vi "Data_Ctrl.vi"() -> ()   [LabVIEW 2019]
uses:
  REV2_Config_Addr.ctl
  <vilib>/event_ctls.llb/eventvkey.ctl
  <vilib>/Instr/_visa.llb/VISA Set IO Buffer Mask.ctl
  <vilib>/Instr/_visa.llb/VISA Flush IO Buffer Mask.ctl
  REV2_Stat_Addr.ctl
  <vilib>/Analysis/1siggen.llb/Ramp Pattern by Samples.vi
  <vilib>/Instr/_visa.llb/VISA Configure Serial Port (Instr).vi
  <vilib>/Analysis/1siggen.llb/Ramp Pattern by Delta.vi
  <vilib>/Analysis/NI_AALBase.lvlib
  <vilib>/ptbypt/NI_PtbyPt.lvlib
panel:
  in  "SAVE":bool
  in  "P0.0002D0.2":bool
  in  "P0.03":bool
  out "VKey":T1
  out "Vbus":dbl(graph)=12.629144668579102
  out "Error count":u64
  out "Array":cluster{"Config Address":T2, dbl}[](array[cluster])=[{"Config Address"=enum."ID", 1.0}, {"Config Address"=enum."Mode", 3.0}, {"Config Address"=enum."Baudrate", 8000000.0}, {"Config Address"=enum."Homing Offset", 0.0}, {"Config Address"=enum."Id P gain", 0.004999999888241291}, {"Config Address"=enum."Id I gain", 0.0010000000474974513}, {"Config Address"=enum."Id D gain", 0.0}, {"Config Address"=enum."Iq P gain", 0.004999999888241291}, {"Config Address"=enum."Iq I gain", 0.0010000000474974513}, {"Config Address"=enum."Iq D gain", 0.0}, {"Config Address"=enum."Velo P gain", 0.4000000059604645}, {"Config Address"=enum."Velo I gain", 0.0010000000474974513}, {"Config Address"=enum."Velo D gain", 0.0}, {"Config Address"=enum."Posi P gain", 0.02500000037252903}, {"Config Address"=enum."Posi I gain", 0.0}, {"Config Address"=enum."Posi D gain", 0.0010000000474974513}, {"Config Address"=enum."DirectForce P", 0.0}, {"Config Address"=enum."DirectForce I", 0.0}, {"Config Address"=enum."DirectForce D", 0.0}, {"Config Address"=enum."Limit Id Max", 50.0}, {"Config Address"=enum."Limit Iq Max", 10.0}, {"Config Address"=enum."Limit Velo Max", 80.0}, {"Config Address"=enum."Limit Posi Min", -131000.0}, {"Config Address"=enum."Limit Posi Max", 131000.0}, {"Config Address"=enum."Voltage Min", 6.0}, {"Config Address"=enum."Voltage Max", 40.0}, {"Config Address"=enum."Low Voltage", 10.0}, {"Config Address"=enum."Temperature Low", 80.0}, {"Config Address"=enum."Temperature High", 100.0}] {"?" format="%#_6f"}
  in  "Read Config":bool
  out "Temperature":cluster{dbl, dbl, dbl}(graph)={25.75, 0.0, 0.0}
  out "ERROR":u8
  out "Iq":cluster{dbl, dbl}(graph)={0.11970416456460953, 0.0}
  out "Id":cluster{dbl, dbl}(graph)={-0.016149107366800308, 0.0}
  out "Theta":cluster{dbl, dbl}(graph)={-51551.1953125, 0.0}
  out "Theta_dot":cluster{dbl, dbl}(graph)={0.09893438220024109, 0.0}
  in  "ID":u8=1
  in  "Read":bool=TRUE
  in  "PID0":bool
  in  "P0.001":bool
  in  "D0.5":bool
  in  "P0.0002":bool
  in  "send sine":bool
  in  "2state":bool
  in  "Chirp":i32(listbox)=2
  out "Waveform Graph":cluster{dbl, dbl, dbl[]}(graph)={0.0, 0.002, array[5500 elements]}
  in  "Sample_rate":dbl=100.0 format="%#_13g"
  out "Theta_LP":sgl=-51551.195
  in  "send chirp":bool
  in  "Enable":bool
  in  "DISABLE":bool
  in  "Write_Mode":bool
  in  "Listbox":i32(listbox)=3
  in  "Write_Limits":bool
  in  "Limits":cluster{"Iq":sgl, "Vel":sgl}={"Iq"=60.0, "Vel"=80.0}
  in  "Goal":T3={"Id"=0.0, "Iq"=0.0, "Posi"=0.0, "Vel"=10.0}
  in  "PID_F":cluster{"P":sgl, "I":sgl, "D":sgl}
  in  "PID_P":cluster{"P":sgl, "I":sgl, "D":sgl}={"P"=0.025, "I"=0.0, "D"=0.001}
  out "Iq":cluster{"Mean":dbl, "Std":dbl}={"Mean"=0.05623460856704041, "Std"=0.04704007521425213} {"Std" format="%.4f"; "Mean" format="%.4f"}
  out "Theta_LP":cluster{"Mean":dbl, "Std":dbl}={"Mean"=-51551.37356875, "Std"=0.30848497864286445}
  out "Id":cluster{"Mean":dbl, "Std":dbl}={"Mean"=0.0007310798299324233, "Std"=0.028296682304707433} {"Std" format="%.4f"; "Mean" format="%.4f"}
  in  "amplitude":dbl=10000.0 format="%#_13g"
  in  "Time":dbl=10.0 format="%#_13g"
  in  "frq_2":dbl=1.0 format="%#_13g"
  in  "frq_1":dbl=1.0 format="%#_13g"
  in  "stop":bool
  in  "Write_Dst":bool
  in  "PID_IqId":cluster{"P":sgl, "I":sgl, "D":sgl}={"P"=0.005, "I"=0.001, "D"=0.0}
  in  "PID_V":cluster{"P":sgl, "I":sgl, "D":sgl}={"P"=0.4, "I"=0.001, "D"=0.0}
  in  "Write_PID":bool
  in  "baud rate":u32=8000000
  in  "Buffer_Size":u32=150000
  in  "VISA resource name":refnum<visa-resource-name>="COM15"
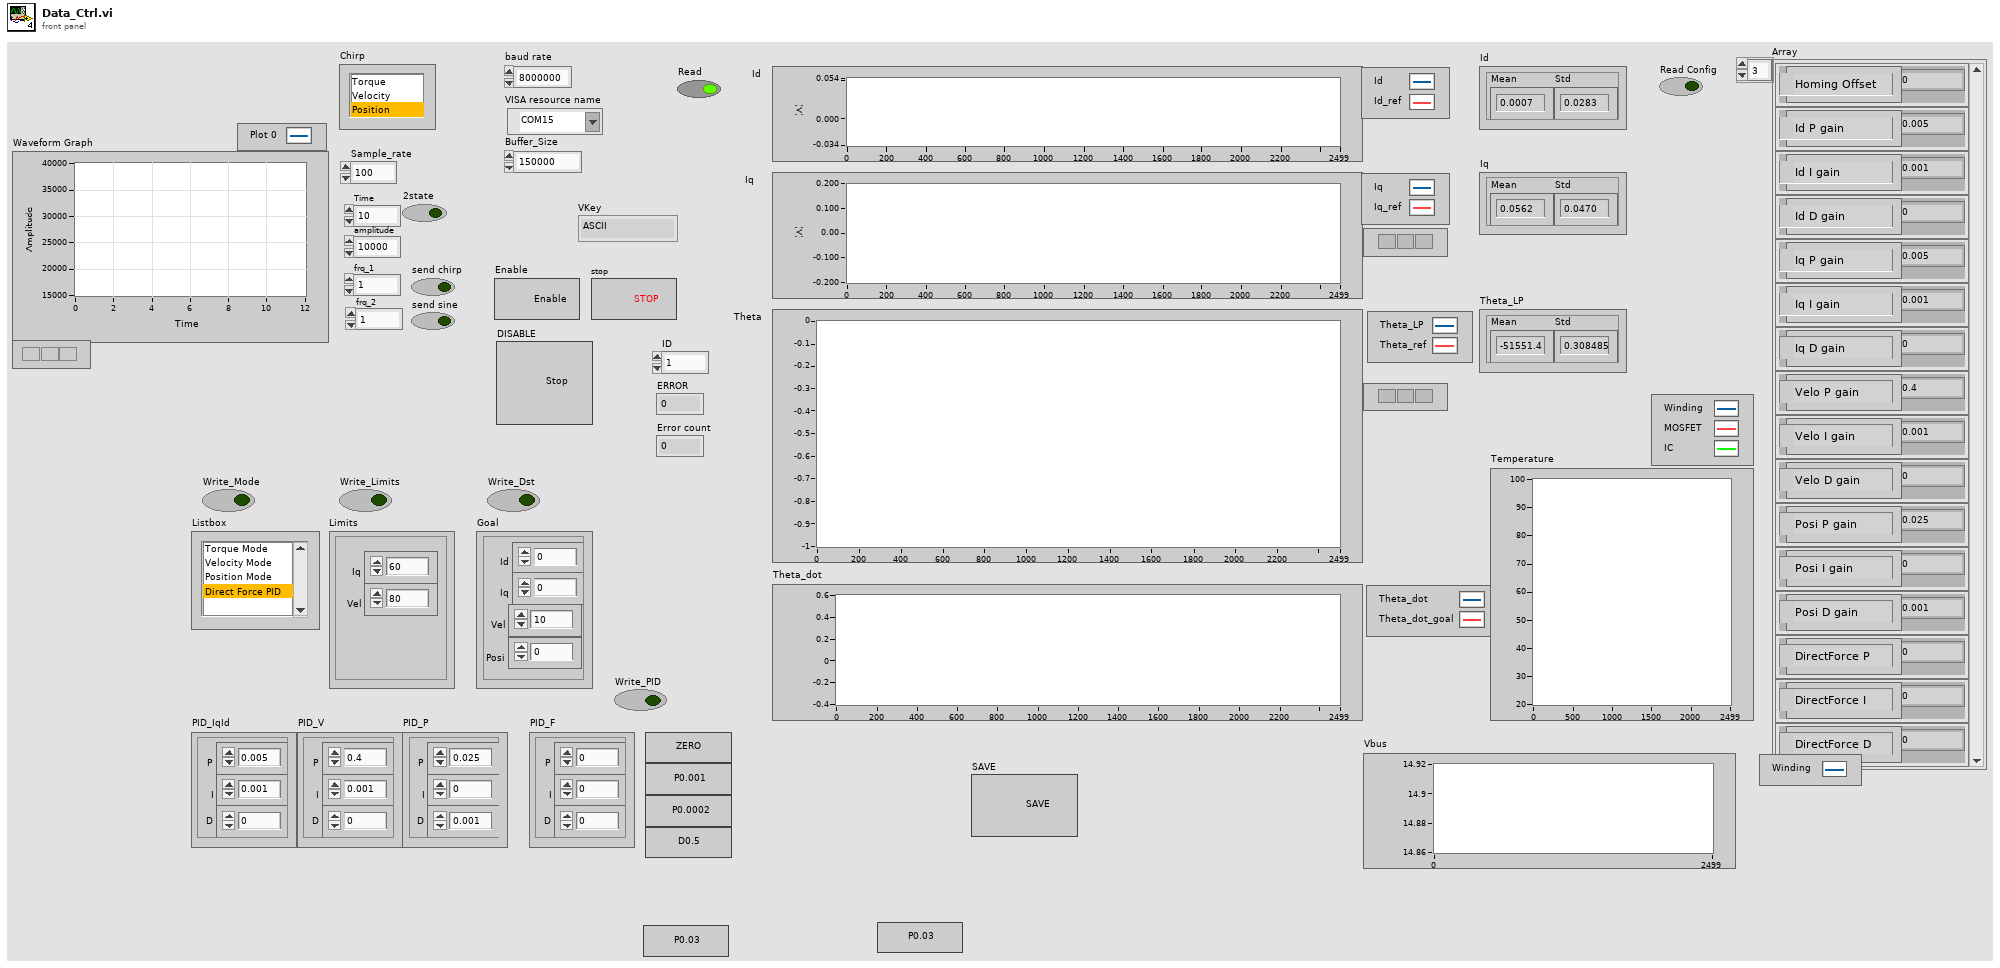
[diagram p1: front panel]
types:
  T1 = typedef "eventvkey.ctl" = enum16{"ASCII", "Enter", "Return", "Shift", "Ctrl", "Alt", "Cmd", "Opt", "Caps", "NumLock", "Clear", "Break", "Up", "Down", "Left", "Right", "Insert", "Delete", "Home", "End", "PageUp", "PageDown", "Escape", "Help", "Pause", "ScrollLock", "F1", "F2", "F3", "F4", "F5", "F6", "F7", "F8", "F9", "F10", "F11", "F12", "F13", "F14", "F15", "F16", "F17", "F18", "F19", "F20", "F21", "F22", "F23", "F24", "Play", "VolumeUp", "VolumeDown", "Mute", "Two Byte Char"}
  T2 = typedef "REV2_Config_Addr.ctl" = enum8{"ID", "Mode", "Baudrate", "Homing Offset", "Id P gain", "Id I gain", "Id D gain", "Iq P gain", "Iq I gain", "Iq D gain", "Velo P gain", "Velo I gain", "Velo D gain", "Posi P gain", "Posi I gain", "Posi D gain", "DirectForce P", "DirectForce I", "DirectForce D", "Limit Id Max", "Limit Iq Max", "Limit Velo Max", "Limit Posi Min", "Limit Posi Max", "Voltage Min", "Voltage Max", "Low Voltage", "Temperature Low", "Temperature High"}
  T3 = cluster{"Id":sgl, "Iq":sgl, "Posi":sgl, "Vel":sgl}
  T4 = typedef "VISA Flush IO Buffer Mask.ctl" = u16
  T5 = typedef "VISA Set IO Buffer Mask.ctl" = u16
  T6 = typedef "REV2_Stat_Addr.ctl" = enum8{"Torque Enable", "Homing Complete", "Goal Id", "Goal Iq", "Goal Velo", "Goal Posi", "Present Id", "Present Iq", "Present Velo", "Present Posi", "Bus Voltage", "Temperature Winding", "Temperature MOSFET", "Temperature IC", "Error Status"}
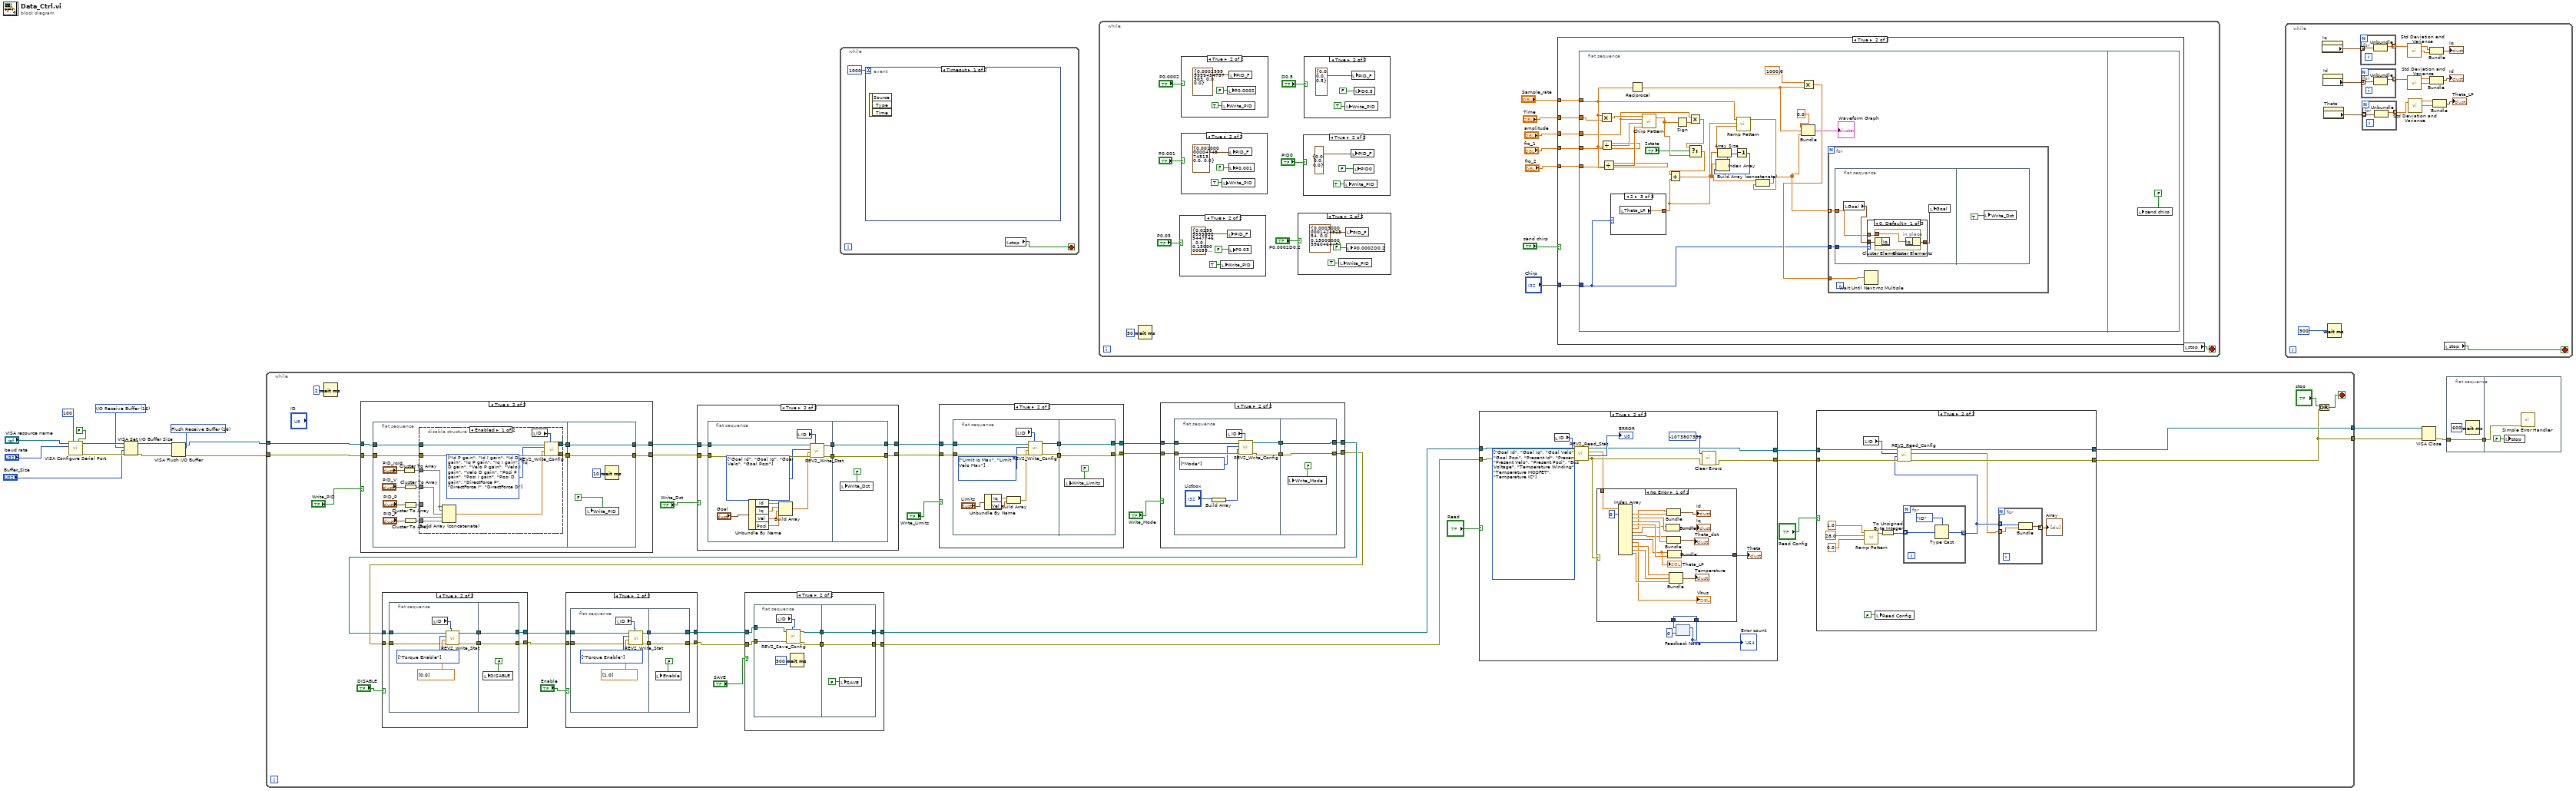
[diagram p0: block diagram]
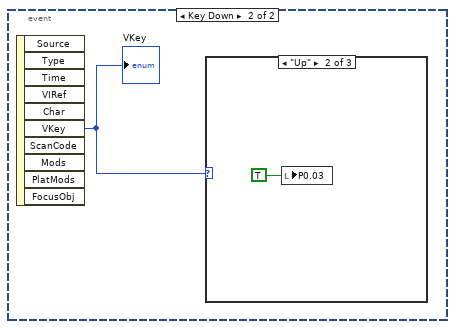
[diagram p2: hidden frame]
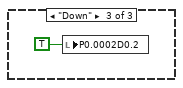
[diagram p4: hidden frame]
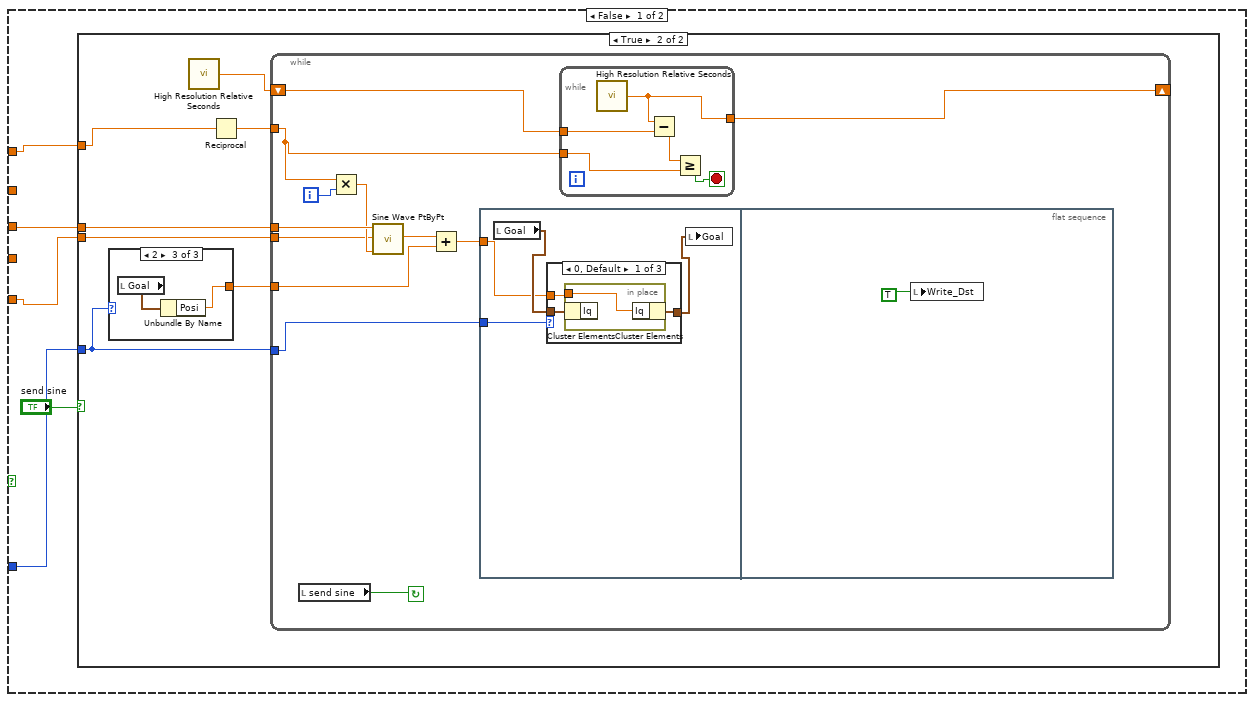
[diagram p11: hidden frame]
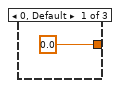
[diagram p13: hidden frame]
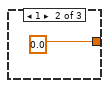
[diagram p14: hidden frame]
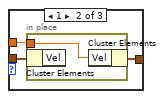
[diagram p15: hidden frame]
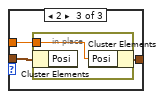
[diagram p16: hidden frame]
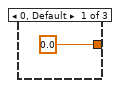
[diagram p17: hidden frame]
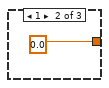
[diagram p18: hidden frame]
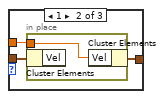
[diagram p19: hidden frame]
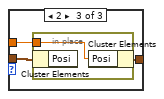
[diagram p20: hidden frame]
diagram:
  w6 = T4 16 items=["Flush Receive Buffer"=16, "Write Transmit Buffer to Device"=32, "Flush Receive Buffer (No I/O)"=64, "Flush Transmit Buffer"=128] ("Mask")
  w10 = T5 16 items=["I/O Receive Buffer"=16, "I/O Transmit Buffer"=32, "I/O Receive and Transmit Buffer"=48] ("Mask")
  n1 = call-poly "VISA Configure Serial Port"("VISA resource name"="VISA resource name", "timeout (10sec)"=u32 100, "Enable Termination\nChar (T)"=FALSE ("Enable Termination\nChar (T)"), "baud rate (9600)"="baud rate") -> ("VISA resource name out"=w12:refnum<visa-resource-name>, "error out"=w11:errorcluster)  [unwired: 10 in]
  n2 = VISA Set I/O Buffer Size(VISA resource name=w12, mask (16)=w10, size (4096)="Buffer_Size", error in (no error)=w11) -> (VISA resource name out=w4:refnum<visa-resource-name>, error out=w5:errorcluster)
  n3 = VISA Flush I/O Buffer(VISA resource name=w4, mask (16)=w6, error in (no error)=w5) -> (VISA resource name out=w1:refnum<visa-resource-name>, error out=w7:errorcluster)
  n4 = while {
    tunnel: w1 -> [w44]
    tunnel: w7 -> [w45]
    tunnel: [w23] -> w15
    tunnel: [w24] -> w14
    stop <- w46 stop-if-true
    n5 = Wait (ms)(milliseconds to wait=u32 2) -> ()  [unwired: 1 out]
    n6 = case shown="True" "Write_PID" {
      tunnel: w44 -> [w228 w235]
      tunnel: w45 -> [w229 w234]
      tunnel: [w229 w233] -> w42
      tunnel: [w228 w232] -> w43
      frame False {
      }
      frame True {
        n7 = flat-sequence {
          tunnel: w235 -> [w247]
          tunnel: w234 -> [w244]
          tunnel: [w246] -> w231
          tunnel: [w245] -> w230
          tunnel: [w267] -> w233
          tunnel: [w268] -> w232
          tunnel: w231 -> [w268]
          tunnel: w230 -> [w267]
          frame #0 {
            n8 = Cluster To Array(cluster="PID_IqId") -> (array=w239:sgl[])
            n9 = Cluster To Array(cluster="PID_V") -> (array=w238:sgl[])
            n10 = Cluster To Array(cluster="PID_P") -> (array=w237:sgl[])
            n11 = Cluster To Array(cluster="PID_F") -> (array=w236:sgl[])
            n12 = disable-structure shown="Enabled" {
              disable-tunnel: w247 -> [w258 w265]
              disable-tunnel: [w257 w264] -> w246
              disable-tunnel: [w255 w262] -> w245
              disable-tunnel: w244 -> [w254 w261]
              disable-tunnel: w239 -> [w252 _]
              disable-tunnel: w238 -> [w251 _]
              disable-tunnel: w237 -> [w250 _]
              disable-tunnel: w236 -> [w249 w259]
              frame Enabled {
                w253 = T2[] [enum."Id P gain", enum."Id I gain", enum."Id D gain", enum."Iq P gain", enum."Iq I gain", enum."Iq D gain", enum."Velo P gain", enum."Velo I gain", enum."Velo D gain", enum."Posi P gain", enum."Posi I gain", enum."Posi D gain", enum."DirectForce P", enum."DirectForce I", enum."DirectForce D"] items=["ID", "Mode", "Baudrate", "Homing Offset", "Id P gain", "Id I gain", "Id D gain", "Iq P gain", "Iq I gain", "Iq D gain", "Velo P gain", "Velo I gain", "Velo D gain", "Posi P gain", "Posi I gain", "Posi D gain", "DirectForce P", "DirectForce I", "DirectForce D", "Limit Id Max", "Limit Iq Max", "Limit Velo Max", "Limit Posi Min", "Limit Posi Max", "Voltage Min", "Voltage Max", "Low Voltage", "Temperature Low", "Temperature High"] ("Config Addr")
                n13 = Build Array (concatenate)(w252, w252, w251, w250, w249) -> (w248:sgl[])
                n14 = local read "ID"() -> (w256:u8)
                n15 = call "REV2_Write_Config.vi"("ID"=w256, "error in (no error)"=w254, "Data"=w248, "Config Addr"=w253, "VISA Refnum in"=w258) -> ("error out"=w255:errorcluster, "VISA Refnum out"=w257:refnum<visa-resource-name>)  [unwired: 5 in]
              }
              frame Disabled {
                w260 = T2[] [enum."DirectForce P", enum."DirectForce I", enum."DirectForce D"] items=["ID", "Mode", "Baudrate", "Homing Offset", "Id P gain", "Id I gain", "Id D gain", "Iq P gain", "Iq I gain", "Iq D gain", "Velo P gain", "Velo I gain", "Velo D gain", "Posi P gain", "Posi I gain", "Posi D gain", "DirectForce P", "DirectForce I", "DirectForce D", "Limit Id Max", "Limit Iq Max", "Limit Velo Max", "Limit Posi Min", "Limit Posi Max", "Voltage Min", "Voltage Max", "Low Voltage", "Temperature Low", "Temperature High"] ("Config Addr")
                n16 = local read "ID"() -> (w263:u8)
                n17 = call "REV2_Write_Config.vi"("ID"=w263, "error in (no error)"=w261, "Data"=w259, "Config Addr"=w260, "VISA Refnum in"=w265) -> ("error out"=w262:errorcluster, "VISA Refnum out"=w264:refnum<visa-resource-name>)  [unwired: 5 in]
              }
            }
          }
          frame #1 {
            n18 = local write "Write_PID"(FALSE ("WriteP_PID")) -> ()
            n19 = Wait (ms)(milliseconds to wait=u32 10) -> ()  [unwired: 1 out]
          }
        }
      }
    }
    n20 = case shown="True" "Write_Dst" {
      tunnel: w42 -> [w206 w212]
      tunnel: w43 -> [w205 w211]
      tunnel: [w206 w210] -> w39
      tunnel: [w205 w209] -> w40
      frame False {
      }
      frame True {
        n21 = flat-sequence {
          tunnel: w212 -> [w218]
          tunnel: w211 -> [w217]
          tunnel: [w216] -> w208
          tunnel: [w215] -> w207
          tunnel: [w225] -> w210
          tunnel: [w226] -> w209
          tunnel: w208 -> [w226]
          tunnel: w207 -> [w225]
          frame #0 {
            w214 = T6[] [enum."Goal Id", enum."Goal Iq", enum."Goal Velo", enum."Goal Posi"] items=["Torque Enable", "Homing Complete", "Goal Id", "Goal Iq", "Goal Velo", "Goal Posi", "Present Id", "Present Iq", "Present Velo", "Present Posi", "Bus Voltage", "Temperature Winding", "Temperature MOSFET", "Temperature IC", "Error Status"] ("Stat Addr")
            n22 = Unbundle By Name("Goal") -> ("Id"=w220:sgl, "Iq"=w221:sgl, "Vel"=w222:sgl, "Posi"=w223:sgl)
            n23 = Build Array(w220, w221, w222, w223) -> (w213:sgl[])
            n24 = local read "ID"() -> (w219:u8)
            n25 = call "REV2_Write_Stat.vi"("ID"=w219, "error in (no error)"=w218, "Data"=w213, "Stat Addr"=w214, "VISA Refnum in"=w217) -> ("error out"=w215:errorcluster, "VISA Refnum out"=w216:refnum<visa-resource-name>)  [unwired: 5 in]
          }
          frame #1 {
            n26 = local write "Write_Dst"(FALSE ("WriteP_PID")) -> ()
          }
        }
      }
    }
    n27 = case shown="True" "Write_Limits" {
      tunnel: w39 -> [w145 w151]
      tunnel: w40 -> [w144 w150]
      tunnel: [w145 w149] -> w36
      tunnel: [w144 w148] -> w37
      frame False {
      }
      frame True {
        n28 = flat-sequence {
          tunnel: w151 -> [w155]
          tunnel: w150 -> [w158]
          tunnel: [w157] -> w147
          tunnel: [w156] -> w146
          tunnel: [w162] -> w149
          tunnel: [w163] -> w148
          tunnel: w147 -> [w163]
          tunnel: w146 -> [w162]
          frame #0 {
            w154 = T2[] [enum."Limit Iq Max", enum."Limit Velo Max"] items=["ID", "Mode", "Baudrate", "Homing Offset", "Id P gain", "Id I gain", "Id D gain", "Iq P gain", "Iq I gain", "Iq D gain", "Velo P gain", "Velo I gain", "Velo D gain", "Posi P gain", "Posi I gain", "Posi D gain", "DirectForce P", "DirectForce I", "DirectForce D", "Limit Id Max", "Limit Iq Max", "Limit Velo Max", "Limit Posi Min", "Limit Posi Max", "Voltage Min", "Voltage Max", "Low Voltage", "Temperature Low", "Temperature High"] ("Config Addr")
            n29 = Unbundle By Name("Limits") -> ("Iq"=w161:sgl, "Vel"=w152:sgl)
            n30 = Build Array(w161, w152) -> (w153:sgl[])
            n31 = local read "ID"() -> (w159:u8)
            n32 = call "REV2_Write_Config.vi"("ID"=w159, "error in (no error)"=w155, "Data"=w153, "Config Addr"=w154, "VISA Refnum in"=w158) -> ("error out"=w156:errorcluster, "VISA Refnum out"=w157:refnum<visa-resource-name>)  [unwired: 5 in]
          }
          frame #1 {
            n33 = local write "Write_Limits"(FALSE ("WriteP_PID")) -> ()
          }
        }
      }
    }
    n34 = case shown="True" "Write_Mode" {
      tunnel: w36 -> [w126 w132]
      tunnel: w37 -> [w125 w131]
      tunnel: [w126 w130] -> w33
      tunnel: [w125 w129] -> w34
      frame False {
      }
      frame True {
        n35 = flat-sequence {
          tunnel: w132 -> [w138]
          tunnel: w131 -> [w139]
          tunnel: [w136] -> w128
          tunnel: [w137] -> w127
          tunnel: [w141] -> w130
          tunnel: [w142] -> w129
          tunnel: w128 -> [w142]
          tunnel: w127 -> [w141]
          frame #0 {
            w135 = T2[] [enum."Mode"] items=["ID", "Mode", "Baudrate", "Homing Offset", "Id P gain", "Id I gain", "Id D gain", "Iq P gain", "Iq I gain", "Iq D gain", "Velo P gain", "Velo I gain", "Velo D gain", "Posi P gain", "Posi I gain", "Posi D gain", "DirectForce P", "DirectForce I", "DirectForce D", "Limit Id Max", "Limit Iq Max", "Limit Velo Max", "Limit Posi Min", "Limit Posi Max", "Voltage Min", "Voltage Max", "Low Voltage", "Temperature Low", "Temperature High"] ("Config Addr")
            n36 = Build Array("Listbox") -> (w134:i32[])
            n37 = local read "ID"() -> (w140:u8)
            n38 = call "REV2_Write_Config.vi"("ID"=w140, "error in (no error)"=w138, "Data"=w134, "Config Addr"=w135, "VISA Refnum in"=w139) -> ("error out"=w137:errorcluster, "VISA Refnum out"=w136:refnum<visa-resource-name>)  [unwired: 5 in]
          }
          frame #1 {
            n39 = local write "Write_Mode"(FALSE ("WriteP_PID")) -> ()
          }
        }
      }
    }
    n40 = case shown="True" "DISABLE" {
      tunnel: w33 -> [w108 w114]
      tunnel: w34 -> [w107 w113]
      tunnel: [w108 w112] -> w30
      tunnel: [w107 w111] -> w31
      frame False {
      }
      frame True {
        n41 = flat-sequence {
          tunnel: w114 -> [w116]
          tunnel: w113 -> [w121]
          tunnel: [w118] -> w110
          tunnel: [w117] -> w109
          tunnel: [w122] -> w112
          tunnel: [w123] -> w111
          tunnel: w110 -> [w123]
          tunnel: w109 -> [w122]
          frame #0 {
            w120 = T6[] [enum."Torque Enable"] items=["Torque Enable", "Homing Complete", "Goal Id", "Goal Iq", "Goal Velo", "Goal Posi", "Present Id", "Present Iq", "Present Velo", "Present Posi", "Bus Voltage", "Temperature Winding", "Temperature MOSFET", "Temperature IC", "Error Status"] ("Stat Addr")
            n42 = local read "ID"() -> (w115:u8)
            n43 = call "REV2_Write_Stat.vi"("ID"=w115, "error in (no error)"=w116, "Data"=dbl[] [0.0], "Stat Addr"=w120, "VISA Refnum in"=w121) -> ("error out"=w117:errorcluster, "VISA Refnum out"=w118:refnum<visa-resource-name>)  [unwired: 5 in]
          }
          frame #1 {
            n44 = local write "DISABLE"(FALSE ("WriteP_PID")) -> ()
          }
        }
      }
    }
    n45 = case shown="True" "Enable" {
      tunnel: w30 -> [w90 w96]
      tunnel: w31 -> [w89 w95]
      tunnel: [w90 w94] -> w19
      tunnel: [w89 w93] -> w21
      frame False {
      }
      frame True {
        n46 = flat-sequence {
          tunnel: w96 -> [w98]
          tunnel: w95 -> [w99]
          tunnel: [w100] -> w92
          tunnel: [w97] -> w91
          tunnel: [w104] -> w94
          tunnel: [w105] -> w93
          tunnel: w92 -> [w105]
          tunnel: w91 -> [w104]
          frame #0 {
            w101 = T6[] [enum."Torque Enable"] items=["Torque Enable", "Homing Complete", "Goal Id", "Goal Iq", "Goal Velo", "Goal Posi", "Present Id", "Present Iq", "Present Velo", "Present Posi", "Bus Voltage", "Temperature Winding", "Temperature MOSFET", "Temperature IC", "Error Status"] ("Stat Addr")
            n47 = local read "ID"() -> (w103:u8)
            n48 = call "REV2_Write_Stat.vi"("ID"=w103, "error in (no error)"=w98, "Data"=dbl[] [1.0], "Stat Addr"=w101, "VISA Refnum in"=w99) -> ("error out"=w97:errorcluster, "VISA Refnum out"=w100:refnum<visa-resource-name>)  [unwired: 5 in]
          }
          frame #1 {
            n49 = local write "Enable"(FALSE ("WriteP_PID")) -> ()
          }
        }
      }
    }
    n50 = case shown="True" "SAVE" {
      tunnel: w21 -> [w51 w57]
      tunnel: w19 -> [w50 w55]
      tunnel: [w51 w56] -> w20
      tunnel: [w50 w54] -> w18
      frame False {
      }
      frame True {
        n51 = flat-sequence {
          tunnel: w57 -> [w63]
          tunnel: w55 -> [w60]
          tunnel: [w61] -> w53
          tunnel: [w59] -> w52
          tunnel: [w65] -> w54
          tunnel: [w66] -> w56
          tunnel: w53 -> [w66]
          tunnel: w52 -> [w65]
          frame #0 {
            n52 = local read "ID"() -> (w62:u8)
            n53 = call "REV2_Save_Config.vi"("ID"=w62, "error in (no error)"=w60, "VISA Refnum in"=w63) -> ("error out"=w59:errorcluster, "VISA Refnum out"=w61:refnum<visa-resource-name>)  [unwired: 7 in]
            n54 = Wait (ms)(milliseconds to wait=u32 500) -> ()  [unwired: 1 out]
          }
          frame #1 {
            n55 = local write "SAVE"(FALSE ("SAVE")) -> ()
          }
        }
      }
    }
    n56 = case shown="True" "Read" {
      tunnel: [w166 w174] -> w25
      tunnel: w18 -> [w165 w179]
      tunnel: w20 -> [w166 w180]
      tunnel: [w165 w171] -> w26
      frame False {
      }
      frame True {
        w177 = T6[] [enum."Goal Id", enum."Goal Iq", enum."Goal Velo", enum."Goal Posi", enum."Present Id", enum."Present Iq", enum."Present Velo", enum."Present Posi", enum."Bus Voltage", enum."Temperature Winding", enum."Temperature MOSFET", enum."Temperature IC"] items=["Torque Enable", "Homing Complete", "Goal Id", "Goal Iq", "Goal Velo", "Goal Posi", "Present Id", "Present Iq", "Present Velo", "Present Posi", "Bus Voltage", "Temperature Winding", "Temperature MOSFET", "Temperature IC", "Error Status"] ("Stat Address")
        n57 = local read "ID"() -> (w178:u8)
        n58 = call "REV2_Read_Stat.vi"("error in (no error)"=w179, "Stat Address"=w177, "ID"=w178, "VISA Refnum in"=w180) -> ("error out"=w172:errorcluster, "ERROR"=→"ERROR":u8, "Data"=w175:dbl[], "VISA Refnum out"=w174:refnum<visa-resource-name>)  [unwired: 4 in]
        n59 = feedback #1(u64 0) -> (w169:u64)
        n60 = case shown="No Error" w172 {
          tunnel: w175 -> [w196 _]
          tunnel: w169 -> [w182 w204]
          tunnel: [w182 w203] -> w168
          tunnel: [w181 w202] -> w167
          frame No Error {
            n61 = Index Array(array=w196, index #1=0 ("index")) -> (element #1=w195:dbl, element #2=w194:dbl, element #3=w193:dbl, element #4=w192:dbl, element #5=w191:dbl, element #6=w190:dbl, element #7=w189:dbl, element #8=w188:dbl, element #9=→"Vbus":dbl, element #10=w184:dbl, element #11=w185:dbl, element #12=w186:dbl)  [unwired: 11 in]
            "Theta_LP" <- w188
            n62 = Bundle(w190, w194) -> (→"Iq":cluster{dbl, dbl})  [unwired: 1 in]
            n63 = Bundle(w189, w193) -> (→"Theta_dot":cluster{dbl, dbl})  [unwired: 1 in]
            n64 = Bundle(w191, w195) -> (→"Id":cluster{dbl, dbl})  [unwired: 1 in]
            n65 = Bundle(w188, w192) -> (w181:cluster{dbl, dbl})  [unwired: 1 in]
            n66 = Bundle(w184, w185, w186) -> (→"Temperature":cluster{dbl, dbl, dbl})  [unwired: 1 in]
          }
          frame Error {
            w201 = nan
            n67 = Increment(x=w204) -> (x+1=w203:u64)
            n68 = Bundle(w201, w201) -> (w202:cluster{dbl, dbl})  [unwired: 1 in]
          }
        }
        "Error count" <- w168
        "Theta" <- w167
        n69 = feedback-in #1(w168) -> ()
        n70 = call <vilib>:"Clear Errors.vi"("error in (no error)"=w172, "specific error code to clear (0: all)"=-1073807339) -> ("error out"=w171:errorcluster)  [unwired: 4 in, 1 out]
      }
    }
    n71 = case shown="True" "Read Config" {
      tunnel: w26 -> [w67 w81]
      tunnel: w25 -> [w68 w80]
      tunnel: [w67 w78] -> w24
      tunnel: [w68 w77] -> w23
      frame False {
      }
      frame True {
        n72 = local read "ID"() -> (w79:u8)
        n73 = call-poly <vilib>:"Ramp Pattern.vi"("start"=0.0, "end"=28.0, "delta"=1.0) -> ("Ramp Pattern"=w73:dbl[])  [unwired: 6 in, 2 out]
        n74 = local write "Read Config"(FALSE ("Read Config")) -> ()
        n75 = To Unsigned Byte Integer(number=w73) -> (unsigned 8bit integer=w72:u8[])
        n76 = for {
          tunnel: w72 -> [w87] mode=indexing
          tunnel: [w86] -> w71 mode=indexing
          n77 = Type Cast(type=REV2_Config_Addr."ID" ("Config Address"), x=w87) -> (*(type *) &x=w86:T2)
        }
        n78 = call "REV2_Read_Config.vi"("error in (no error)"=w81, "Config Address"=w71, "ID"=w79, "VISA Refnum in"=w80) -> ("error out"=w78:errorcluster, "Data"=w70:dbl[], "VISA Refnum out"=w77:refnum<visa-resource-name>)  [unwired: 4 in, 1 out]
        n79 = for {
          tunnel: w71 -> [w85] mode=indexing
          tunnel: w70 -> [w84] mode=indexing
          tunnel: [w83] -> w69 mode=indexing
          n80 = Bundle("Config Address"=w85, w84) -> (w83:cluster{"Config Address":T2, dbl})  [unwired: 1 in]
        }
        "Array" <- w69
      }
    }
    n81 = Or(x="stop", y=w24) -> (x .or. y?=w46:bool)
  }
  n82 = while {
    stop <- w271 stop-if-true
    n83 = event shown="[0] Timeout" {
      selector: _ -> [_ _]
      dyn-events: _ -> [_ _]
      timeout: 1000 -> [_ _]
      event Timeout {
        n84 = event-data() -> ()  [unwired: 1 in, 3 out]
      }
      event Key Down {
        n85 = event-data() -> ("VKey"=w272:T1)  [unwired: 1 in, 9 out]
        "VKey" <- w272
        n86 = case shown="\"Up\"" w272 {
          frame "ASCII", Default {
          }
          frame "Up" {
            n87 = local write "P0.03"(TRUE ("P0.0002")) -> ()
          }
          frame "Down" {
            n88 = local write "P0.0002D0.2"(TRUE ("P0.0002")) -> ()
          }
        }
      }
    }
    n89 = local read "stop"() -> (w271:bool)
  }
  n90 = while {
    stop <- w289 stop-if-true
    n91 = Wait (ms)(milliseconds to wait=u32 50) -> ()  [unwired: 1 out]
    n92 = case shown="True" "P0.03" {
      frame False {
      }
      frame True {
        n93 = local write "Write_PID"(TRUE ("Write_PID")) -> ()
        n94 = local write "PID_F"(cluster{"P":sgl, "I":sgl, "D":sgl} {"P"=0.03, "I"=0.0, "D"=0.15} ("PID_F 2")) -> ()
        n95 = local write "P0.03"(FALSE ("P0.0002")) -> ()
      }
    }
    n96 = case shown="True" "P0.001" {
      frame False {
      }
      frame True {
        n97 = local write "Write_PID"(TRUE ("Write_PID")) -> ()
        n98 = local write "PID_F"(cluster{"P":sgl, "I":sgl, "D":sgl} {"P"=0.001, "I"=0.0, "D"=0.0} ("PID_F 2")) -> ()
        n99 = local write "P0.001"(FALSE ("P0.0002")) -> ()
      }
    }
    n100 = case shown="True" "P0.0002" {
      frame False {
      }
      frame True {
        n101 = local write "Write_PID"(TRUE ("Write_PID")) -> ()
        n102 = local write "P0.0002"(FALSE ("P0.0002")) -> ()
        n103 = local write "PID_F"(cluster{"P":sgl, "I":sgl, "D":sgl} {"P"=0.0002, "I"=0.0, "D"=0.0} ("PID_F 2")) -> ()
      }
    }
    n104 = case shown="True" "P0.0002D0.2" {
      frame False {
      }
      frame True {
        n105 = local write "Write_PID"(TRUE ("Write_PID")) -> ()
        n106 = local write "PID_F"(cluster{"P":sgl, "I":sgl, "D":sgl} {"P"=0.0003, "I"=0.0, "D"=0.15} ("PID_F 2")) -> ()
        n107 = local write "P0.0002D0.2"(FALSE ("P0.0002")) -> ()
      }
    }
    n108 = case shown="True" "PID0" {
      frame False {
      }
      frame True {
        n109 = local write "Write_PID"(TRUE ("Write_PID")) -> ()
        n110 = local write "PID_F"(cluster{"P":sgl, "I":sgl, "D":sgl} {"P"=0.0, "I"=0.0, "D"=0.0} ("PID_F 2")) -> ()
        n111 = local write "PID0"(FALSE ("P0.0002")) -> ()
      }
    }
    n112 = case shown="True" "D0.5" {
      frame False {
      }
      frame True {
        n113 = local write "Write_PID"(TRUE ("Write_PID")) -> ()
        n114 = local write "PID_F"(cluster{"P":sgl, "I":sgl, "D":sgl} {"P"=0.0, "I"=0.0, "D"=0.5} ("PID_F 2")) -> ()
        n115 = local write "D0.5"(FALSE ("P0.0002")) -> ()
      }
    }
    n116 = case shown="True" "send chirp" {
      tunnel: "Chirp" -> [w309 w363]
      tunnel: "Sample_rate" -> [w311 w362]
      tunnel: "Time" -> [_ w361]
      tunnel: "amplitude" -> [w310 w360]
      tunnel: "frq_1" -> [_ w359]
      tunnel: "frq_2" -> [w308 w358]
      frame False {
        n117 = case shown="True" "send sine" {
          tunnel: w311 -> [_ w315]
          tunnel: w310 -> [_ w316]
          tunnel: w309 -> [_ w318]
          tunnel: w308 -> [_ w319]
          frame False {
          }
          frame True {
            n118 = case shown="2" w318 {
              tunnel: [0.0 ("x") 0.0 ("x") w322] -> w317
              frame 0, Default {
              }
              frame 1 {
              }
              frame 2 {
                n119 = local read "Goal"() -> (w323:T3)
                n120 = Unbundle By Name(w323) -> ("Posi"=w322:sgl)
              }
            }
            n121 = call <vilib>:"High Resolution Relative Seconds.vi"() -> ("relative seconds"=w313:dbl)
            n122 = Reciprocal(x=w315) -> (1/x=w314:dbl)
            n123 = while {
              tunnel: w316 -> [w335]
              tunnel: w318 -> [w328]
              tunnel: w319 -> [w332]
              tunnel: w317 -> [w327]
              tunnel: w314 -> [w324]
              shift-right: [w326] -> _
              shift-left: w313 -> [w325]
              i -> [w334]
              stop <- w331 continue-if-true
              n124 = local read "send sine"() -> (w331:bool)
              n125 = Multiply(x=w324, y=w334) -> (x*y=w333:dbl)
              n126 = call <vilib>:"Sine Wave PtByPt.vi"("time"=w333, "frequency"=w332, "amplitude"=w335) -> ("sine wave"=w330:dbl)  [unwired: 1 in]
              n127 = Add(x=w330, y=w327) -> (x+y=w329:dbl)
              n128 = flat-sequence {
                tunnel: w329 -> [w343]
                tunnel: w328 -> [w342]
                frame #0 {
                  n129 = local read "Goal"() -> (w344:T3)
                  n130 = case shown="0, Default" w342 {
                    tunnel: w344 -> [w347 w351 w355]
                    tunnel: w343 -> [w345 w349 w354]
                    tunnel: [w346 w350 w353] -> w341
                    frame 0, Default {
                      n131 = in-place {
                        in-place-border: w345 -> [w348]
                        n132 = in-place-cluster #2(w347) -> ()  [unwired: 1 out]
                        n133 = in-place-cluster #2("Iq"=w348) -> (w346:T3)
                      }
                    }
                    frame 1 {
                      n134 = in-place {
                        in-place-border: w349 -> [w352]
                        n135 = in-place-cluster #3(w351) -> ()  [unwired: 1 out]
                        n136 = in-place-cluster #3("Vel"=w352) -> (w350:T3)
                      }
                    }
                    frame 2 {
                      n137 = in-place {
                        in-place-border: w354 -> [w356]
                        n138 = in-place-cluster #4(w355) -> ()  [unwired: 1 out]
                        n139 = in-place-cluster #4("Posi"=w356) -> (w353:T3)
                      }
                    }
                  }
                  n140 = local write "Goal"(w341) -> ()
                }
                frame #1 {
                  n141 = local write "Write_Dst"(TRUE ("Write_Dst")) -> ()
                }
              }
              n142 = while {
                tunnel: [w340] -> w326
                tunnel: w325 -> [w339]
                tunnel: w324 -> [w336]
                stop <- w337 stop-if-true
                n143 = call <vilib>:"High Resolution Relative Seconds.vi"() -> ("relative seconds"=w340:dbl)
                n144 = Subtract(x=w340, y=w339) -> (x-y=w338:dbl)
                n145 = Greater Or Equal?(x=w338, y=w336) -> (x >= y?=w337:bool)
              }
            }
          }
        }
      }
      frame True {
        n146 = flat-sequence {
          tunnel: w363 -> [w381]
          tunnel: w362 -> [w368]
          tunnel: w361 -> [w367]
          tunnel: w360 -> [w366]
          tunnel: w359 -> [w365]
          tunnel: w358 -> [w364]
          frame #0 {
            n147 = Multiply(x=w368, y=w367) -> (x*y=w386:dbl)
            n148 = Divide(x=w365, y=w368) -> (x/y=w388:dbl)
            n149 = Divide(x=w364, y=w368) -> (x/y=w387:dbl)
            n150 = case shown="2" w381 {
              tunnel: [0.0 ("x") 0.0 ("x") w392] -> w373
              frame 0, Default {
              }
              frame 1 {
              }
              frame 2 {
                n151 = local read "Theta_LP"() -> (w392:sgl)
              }
            }
            n152 = Reciprocal(x=w368) -> (1/x=w385:dbl)
            n153 = call <vilib>:"Chirp Pattern.vi"("f2"=w387, "f1"=w388, "amplitude"=w366, "samples"=w386) -> ("Chirp Pattern"=w378:dbl[])  [unwired: 1 out]
            n154 = Sign(1:w378) -> (0:w380:dbl[])
            n155 = Multiply(x=w366, y=w380) -> (x*y=w379:dbl[])
            n156 = Select(t=w379, s="2state", f=w378) -> (s? t:f=w377:dbl[])
            n157 = Add(x=w377, y=w373) -> (x+y=w371:dbl[])
            n158 = Array Size(array=w371) -> (size(s)=w375:i32)
            n159 = Decrement(x=w375) -> (x-1=w374:i32)
            n160 = Index Array(array=w371, index=w374) -> (element=w372:dbl)
            n161 = call-poly <vilib>:"Ramp Pattern.vi"("start"=w372, "end"=w373, "samples"=w368) -> ("Ramp Pattern"=w370:dbl[])  [unwired: 7 in, 1 out]
            n162 = Build Array (concatenate)(w371, w370) -> (w369:dbl[])
            n163 = Multiply(x=1000.0, y=w385) -> (x*y=w383:dbl)
            n164 = Bundle(0.0, w385, w369) -> (→"Waveform Graph":cluster{dbl, dbl, dbl[]})  [unwired: 1 in]
            n165 = for {
              tunnel: w369 -> [w395] mode=indexing
              tunnel: w383 -> [w394]
              tunnel: w381 -> [w393]
              n166 = flat-sequence {
                tunnel: w395 -> [w398]
                tunnel: w393 -> [w397]
                frame #0 {
                  n167 = local read "Goal"() -> (w399:T3)
                  n168 = case shown="0, Default" w397 {
                    tunnel: w399 -> [w402 w406 w410]
                    tunnel: w398 -> [w400 w404 w409]
                    tunnel: [w401 w405 w408] -> w396
                    frame 0, Default {
                      n169 = in-place {
                        in-place-border: w400 -> [w403]
                        n170 = in-place-cluster #5(w402) -> ()  [unwired: 1 out]
                        n171 = in-place-cluster #5("Iq"=w403) -> (w401:T3)
                      }
                    }
                    frame 1 {
                      n172 = in-place {
                        in-place-border: w404 -> [w407]
                        n173 = in-place-cluster #6(w406) -> ()  [unwired: 1 out]
                        n174 = in-place-cluster #6("Vel"=w407) -> (w405:T3)
                      }
                    }
                    frame 2 {
                      n175 = in-place {
                        in-place-border: w409 -> [w411]
                        n176 = in-place-cluster #7(w410) -> ()  [unwired: 1 out]
                        n177 = in-place-cluster #7("Posi"=w411) -> (w408:T3)
                      }
                    }
                  }
                  n178 = local write "Goal"(w396) -> ()
                }
                frame #1 {
                  n179 = local write "Write_Dst"(TRUE ("Write_Dst")) -> ()
                }
              }
              n180 = Wait Until Next ms Multiple(millisecond multiple=w394) -> ()  [unwired: 1 out]
            }
          }
          frame #1 {
            n181 = local write "send chirp"(FALSE ("send chirp")) -> ()
          }
        }
      }
    }
    n182 = local read "stop"() -> (w289:bool)
  }
  n183 = while {
    stop <- w416 stop-if-true
    n184 = property on="Iq" class="WFChart (strict)"() -> ("History Data"=w430:cluster{dbl, dbl}[])  [unwired: 2 in, 2 out]
    n185 = property on="Id" class="WFChart (strict)"() -> ("History Data"=w429:cluster{dbl, dbl}[])  [unwired: 2 in, 2 out]
    n186 = property on="Theta" class="WFChart (strict)"() -> ("History Data"=w414:cluster{dbl, dbl}[])  [unwired: 2 in, 2 out]
    n187 = Wait (ms)(milliseconds to wait=u32 500) -> ()  [unwired: 1 out]
    n188 = for {
      tunnel: w430 -> [w436] mode=indexing
      tunnel: [w435] -> w428 mode=indexing
      n189 = Unbundle(w436) -> (w435:dbl)  [unwired: 1 out]
    }
    n190 = for {
      tunnel: w429 -> [w434] mode=indexing
      tunnel: [w433] -> w426 mode=indexing
      n191 = Unbundle(w434) -> (w433:dbl)  [unwired: 1 out]
    }
    n192 = for {
      tunnel: w414 -> [w431] mode=indexing
      tunnel: [w432] -> w427 mode=indexing
      n193 = Unbundle(w431) -> (w432:dbl)  [unwired: 1 out]
    }
    n194 = call <vilib>:"Std Deviation and Variance.vi"("X"=w428) -> ("mean"=w425:dbl, "standard deviation"=w424:dbl)  [unwired: 1 in, 1 out]
    n195 = call <vilib>:"Std Deviation and Variance.vi"("X"=w426) -> ("mean"=w419:dbl, "standard deviation"=w418:dbl)  [unwired: 1 in, 1 out]
    n196 = call <vilib>:"Std Deviation and Variance.vi"("X"=w427) -> ("mean"=w420:dbl, "standard deviation"=w421:dbl)  [unwired: 1 in, 1 out]
    n197 = Bundle("mean"=w419, "standard deviation"=w418) -> (→"Id":cluster{"mean":dbl, "standard deviation":dbl})  [unwired: 1 in]
    n198 = Bundle("mean"=w425, "standard deviation"=w424) -> (→"Iq":cluster{"mean":dbl, "standard deviation":dbl})  [unwired: 1 in]
    n199 = Bundle("mean"=w420, "standard deviation"=w421) -> (→"Theta_LP":cluster{"mean":dbl, "standard deviation":dbl})  [unwired: 1 in]
    n200 = local read "stop"() -> (w416:bool)
  }
  n201 = VISA Close(VISA resource name=w15, error in (no error)=w14) -> (error out=w3:errorcluster)
  n202 = flat-sequence {
    tunnel: w3 -> [w438]
    tunnel: [w438] -> w2
    tunnel: w2 -> [w439]
    frame #0 {
      n203 = Wait (ms)(milliseconds to wait=u32 600) -> ()  [unwired: 1 out]
    }
    frame #1 {
      n204 = local write "stop"(FALSE ("stop")) -> ()
      n205 = call <vilib>:"Simple Error Handler.vi"("error in (no error)"=w439) -> ()  [unwired: 4 in, 5 out]
    }
  }
